vi "testBasic Event Tetst.vi"(8 "error in (no error)":errorcluster, 11 "TestCase in":refnum<class "Event Test Template Examples.lvclass">) -> (0 "error out":errorcluster, 3 "TestCase out":refnum<class "Event Test Template Examples.lvclass">)   [LabVIEW 2015, in "Event Test Template Examples.lvclass"]
uses:
  Event Test Template Examples.lvclass
panel:
  in  "Numeric":dbl
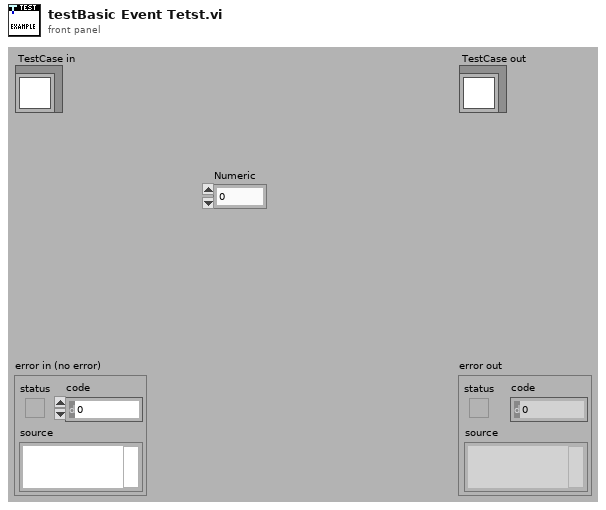
[diagram p1: front panel]
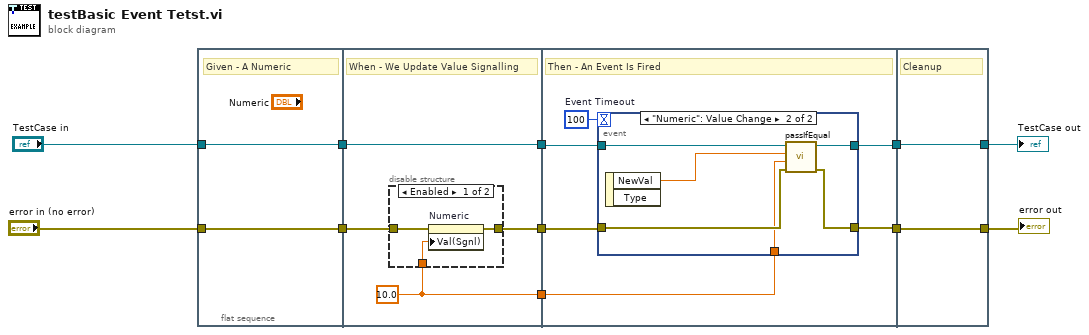
[diagram p0: block diagram]
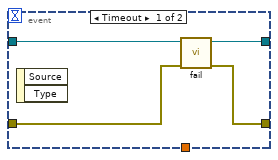
[diagram p3: hidden frame]
diagram:
  n1 = flat-sequence {
    tunnel: "error in (no error)" -> [w12]
    tunnel: "TestCase in" -> [w13]
    tunnel: [w13] -> w7
    tunnel: [w12] -> w6
    tunnel: [w17] -> w5
    tunnel: [w15] -> w4
    tunnel: w7 -> [w17]
    tunnel: w6 -> [w16]
    tunnel: [w14] -> w3
    tunnel: [w26] -> w2
    tunnel: [w23] -> w1
    tunnel: w5 -> [w25]
    tunnel: w4 -> [w24]
    tunnel: w3 -> [w22]
    tunnel: [w38] -> w10
    tunnel: [w39] -> w8
    tunnel: w2 -> [w39]
    tunnel: w1 -> [w38]
    frame #0 {
      # "Given - A Numeric"
    }
    frame #1 {
      w14 = 10.0 ("Value (Signaling)")
      # "When - We Update Value Signalling"
      n2 = disable-structure shown="Enabled" {
        disable-tunnel: w16 -> [w20 w21]
        disable-tunnel: [w19 w21] -> w15
        disable-tunnel: w14 -> [w18 _]
        frame Enabled {
          n3 = property on="Numeric" class="DigNum (strict)"(error in=w20, "Val(Sgnl)"=w18) -> (error out=w19:errorcluster)  [unwired: 1 in, 1 out]
        }
        frame Disabled {
        }
      }
    }
    frame #2 {
      w27 = 100  # Event Timeout
      # "Then - An Event Is Fired"
      n4 = event shown="[1] \"Numeric\": Value Change" {
        selector: _ -> [_ _]
        dyn-events: _ -> [_ _]
        timeout: w27 -> [_ _]
        tunnel: w25 -> [w31 w37]
        tunnel: [w30 w36] -> w26
        tunnel: [w29 w35] -> w23
        tunnel: w24 -> [w28 w34]
        tunnel: w22 -> [_ w33]
        event Timeout {
          n5 = event-data() -> ()  [unwired: 1 in, 2 out]
          n6 = call-dynamic "fail.vi"("error in (no error)"=w28, "TestCase in"=w31) -> ("error out"=w29:errorcluster, "TestCase out"=w30:refnum<class "Event Test Template Examples.lvclass">)  [unwired: 8 in]
        }
        event "Numeric": Value Change {
          n7 = event-data() -> ("NewVal"=w32:dbl)  [unwired: 1 in, 1 out]
          n8 = call-dynamic "passIfEqual.vi"("error in (no error)"=w34, "y"=w33, "x"=w32, "TestCase in"=w37) -> ("error out"=w35:errorcluster, "TestCase out"=w36:refnum<class "Event Test Template Examples.lvclass">)  [unwired: 6 in]
        }
      }
    }
    frame #3 {
      # "Cleanup"
    }
  }
  "error out" <- w10
  "TestCase out" <- w8
